vi "Untitled 1.vi"() -> ()   [LabVIEW 2025]
uses:
  <vilib>/vision/NI_Vision_Development_Module.lvlib
panel:
  out "x-y":dbl
  out "end diff":dbl
  out "error out":errorcluster
  out "Image":T1(plugin-control)
  out "GB/s 2":dbl
  out "GB/s":dbl
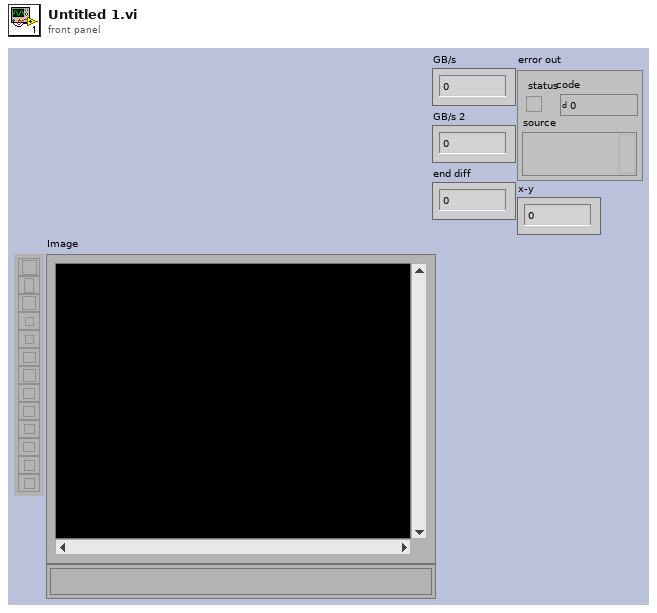
[diagram p1: front panel]
types:
  T1 = typedef "IMAQ Image.ctl" = refnum<image>
  T2 = typedef "Rendezvous RefNum" = refnum<k1>
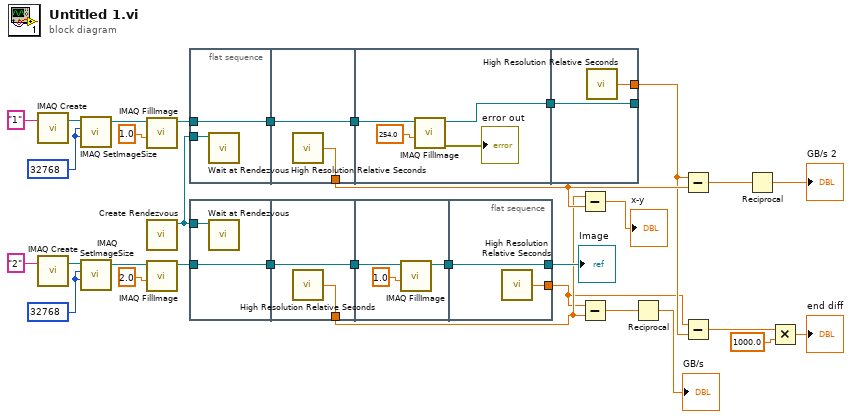
[diagram p0: block diagram]
diagram:
  w19 = 32768 ("X Resolution")
  w30 = 32768 ("X Resolution")
  n1 = call "IMAQ Create"("Image Name"="1") -> ("New Image"=w18:T1)  [unwired: 4 in, 1 out]
  n2 = call "IMAQ Create"("Image Name"="2") -> ("New Image"=w31:T1)  [unwired: 4 in, 1 out]
  n3 = call "IMAQ SetImageSize"("Y Resolution"=w19, "X Resolution"=w19, "Image"=w18) -> ("Image Out"=w20:T1)  [unwired: 2 in, 1 out]
  n4 = call "IMAQ SetImageSize"("Y Resolution"=w30, "X Resolution"=w30, "Image"=w31) -> ("Image Out"=w29:T1)  [unwired: 2 in, 1 out]
  n5 = call "IMAQ FillImage"("Pixel Value (U8, U16, I16, Float)"=sgl 1.0, "Image"=w20) -> ("Image Out"=w21:T1)  [unwired: 8 in, 1 out]
  n6 = call <vilib>:"Create Rendezvous.vi"() -> ("rendezvous"=w14:T2)  [unwired: 5 in, 2 out]
  n7 = call "IMAQ FillImage"("Pixel Value (U8, U16, I16, Float)"=sgl 2.0, "Image"=w29) -> ("Image Out"=w28:T1)  [unwired: 8 in, 1 out]
  n8 = flat-sequence {
    tunnel: w21 -> [w34]
    tunnel: [w34] -> w16
    tunnel: w14 -> [w33]
    tunnel: [w36] -> w24
    tunnel: [w35] -> w8
    tunnel: w16 -> [w36]
    tunnel: w24 -> [w40]
    tunnel: [w39] -> w10
    tunnel: [w42] -> w6
    tunnel: [w41] -> _
    tunnel: w10 -> [w41]
    frame #0 {
      n9 = call <vilib>:"Wait at Rendezvous.vi"("rendezvous"=w33) -> ()  [unwired: 4 in, 3 out]
    }
    frame #1 {
      n10 = call <vilib>:"High Resolution Relative Seconds.vi"() -> ("relative seconds"=w35:dbl)
    }
    frame #2 {
      n11 = call "IMAQ FillImage"("Pixel Value (U8, U16, I16, Float)"=sgl 254.0, "Image"=w40) -> ("error out"=→"error out":errorcluster, "Image Out"=w39:T1)  [unwired: 8 in]
    }
    frame #3 {
      n12 = call <vilib>:"High Resolution Relative Seconds.vi"() -> ("relative seconds"=w42:dbl)
    }
  }
  n13 = flat-sequence {
    tunnel: w28 -> [w44]
    tunnel: [w44] -> w15
    tunnel: w14 -> [w43]
    tunnel: [w46] -> w27
    tunnel: [w45] -> w7
    tunnel: w15 -> [w46]
    tunnel: w27 -> [w49]
    tunnel: [w48] -> w11
    tunnel: [w51] -> w1
    tunnel: [w50] -> w9
    tunnel: w11 -> [w50]
    frame #0 {
      n14 = call <vilib>:"Wait at Rendezvous.vi"("rendezvous"=w43) -> ()  [unwired: 4 in, 3 out]
    }
    frame #1 {
      n15 = call <vilib>:"High Resolution Relative Seconds.vi"() -> ("relative seconds"=w45:dbl)
    }
    frame #2 {
      n16 = call "IMAQ FillImage"("Pixel Value (U8, U16, I16, Float)"=sgl 1.0, "Image"=w49) -> ("Image Out"=w48:T1)  [unwired: 8 in, 1 out]
    }
    frame #3 {
      n17 = call <vilib>:"High Resolution Relative Seconds.vi"() -> ("relative seconds"=w51:dbl)
    }
  }
  n18 = Subtract(x=w7, y=w8) -> (x-y=→"x-y":dbl)
  n19 = Subtract(x=w1, y=w7) -> (x-y=w26:dbl)
  n20 = Reciprocal(x=w26) -> (1/x=→"GB/s":dbl)
  n21 = Subtract(x=w6, y=w8) -> (x-y=w22:dbl)
  n22 = Subtract(x=w1, y=w6) -> (x-y=w5:dbl)
  n23 = Reciprocal(x=w22) -> (1/x=→"GB/s 2":dbl)
  n24 = Multiply(x=w5, y=1000.0) -> (x*y=→"end diff":dbl)
  "Image" <- w9
